vi "Read Initial Frequency and Phase.vi"(8 "error in (no error)":errorcluster, 11 "SV Signal in":refnum<class "SV Signal.lvclass">) -> (0 "error out":errorcluster, 1 "initial phase":dbl, 2 "initial frequency":dbl, 3 "SV Signal out":refnum<class "SV Signal.lvclass">, 4 "found?":bool)   [LabVIEW 2017, in "SV Signal.lvclass"]
uses:
  <vilib>/addons/_NISVFA/_Generation/Signal Generation/SV Signal/SV Signal.lvclass
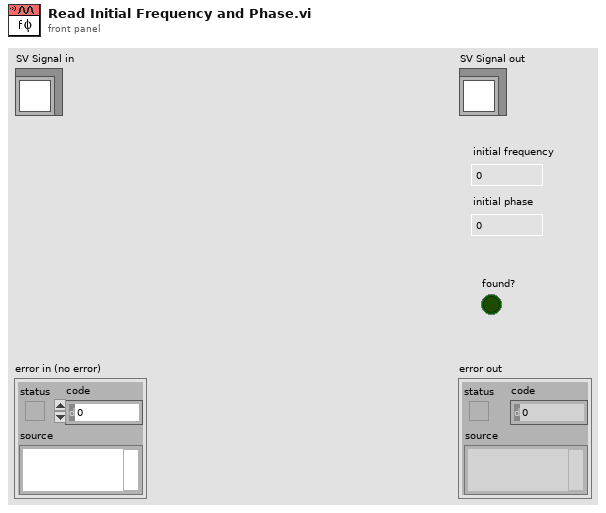
[diagram p1: front panel]
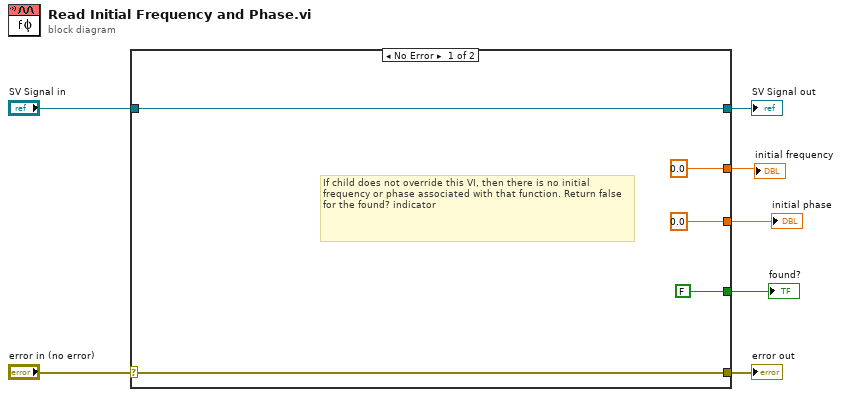
[diagram p0: block diagram]
diagram:
  n1 = case shown="No Error" "error in (no error)" {
    selector: "error in (no error)" -> [w11 w14]
    tunnel: [w11 w14] -> w6
    tunnel: [w12 w13] -> w4
    tunnel: "SV Signal in" -> [w12 w13]
    tunnel: [FALSE ("found?") _] -> w3
    tunnel: [0.0 ("initial phase") _] -> w2
    tunnel: [0.0 ("initial frequency") _] -> w1
    frame No Error {
      # "If child does not override this VI, then there is no initial frequency or phase associated with that function. Return false for the found? indicator"
    }
    frame Error {
    }
  }
  "error out" <- w6
  "SV Signal out" <- w4
  "initial frequency" <- w1
  "initial phase" <- w2
  "found?" <- w3
